vi "World To Display.vi"(10 "World Position":refnum<class "Vector 2D.lvclass">, 11 "Camera in":refnum<class "Camera.lvclass">) -> (3 "Display Position":refnum<class "Vector 2D.lvclass">)   [LabVIEW 2021, in "Camera.lvclass"]
uses:
  Camera.lvclass
  Re-use Libraries/Vector 2D/Vector 2D.lvclass
  Camera.lvclass/Camera.ctl
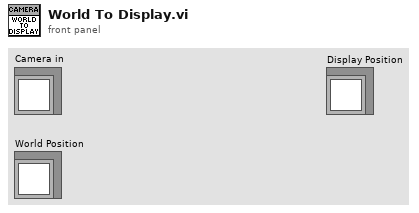
[diagram p1: front panel]
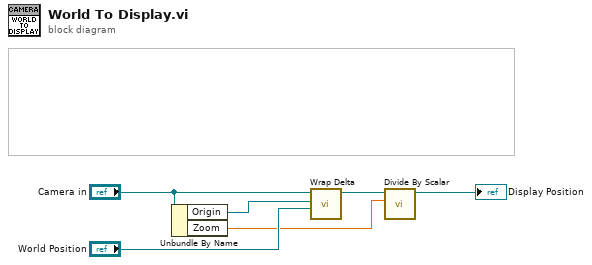
[diagram p0: block diagram]
diagram:
  n1 = Unbundle By Name("Camera in") -> ("Origin"=w5:refnum<class "Vector 2D.lvclass">, "Zoom"=w1:sgl)
  n2 = call "Wrap Delta.vi"("B"="World Position", "A"=w5, "Camera in"="Camera in") -> ("Wrapped Delta"=w3:refnum<class "Vector 2D.lvclass">)  [unwired: 8 in]
  n3 = call "Divide By Scalar.vi"("x"=w1, "A"=w3) -> ("Ax"=→"Display Position":refnum<class "Vector 2D.lvclass">)  [unwired: 9 in]
